vi "Format Error.vi"(5 "show call chain? (True)":bool=TRUE, 7 "error code (402842)":i32=402842, 8 "error in (no error)":errorcluster, 10 "message part 2":string, 11 "error message":string) -> (0 "error out":errorcluster)   [LabVIEW 2024, in "JSONtext.lvlib"]
uses:
  JSONtext.lvlib
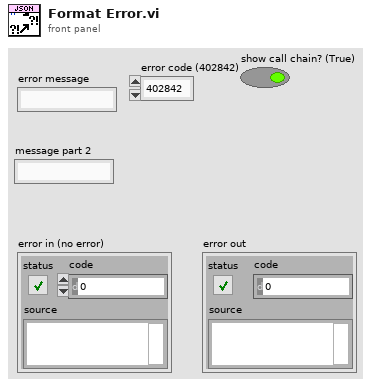
[diagram p1: front panel]
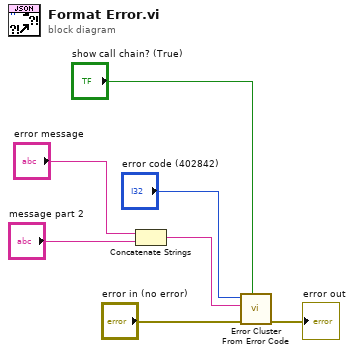
[diagram p0: block diagram]
diagram:
  n1 = Concatenate Strings("error message", "message part 2") -> (w2:string)
  n2 = call "Error Cluster From Error Code.vi"("show call chain? (False)"="show call chain? (True)", "error in (no error)"="error in (no error)", "error message (\"\")"=w2, "error code (0)"="error code (402842)") -> ("error out"=→"error out":errorcluster)  [unwired: 5 in]
